vi "Encode.vi"(8 "error in (no error)":errorcluster, 11 "ISO 14443 B DOWN in":refnum<class "ISO 14443 B DOWN.lvclass">) -> (0 "error out":errorcluster, 3 "ISO 14443 B DOWN out":refnum<class "ISO 14443 B DOWN.lvclass">)   [LabVIEW 2019, in "ISO 14443 B DOWN.lvclass"]
uses:
  ISO 14443 B DOWN.lvclass
  TypeDef/Store.ctl
  ISO 14443 B DOWN.lvclass/ISO 14443 B DOWN.ctl
  RFID system.lvclass
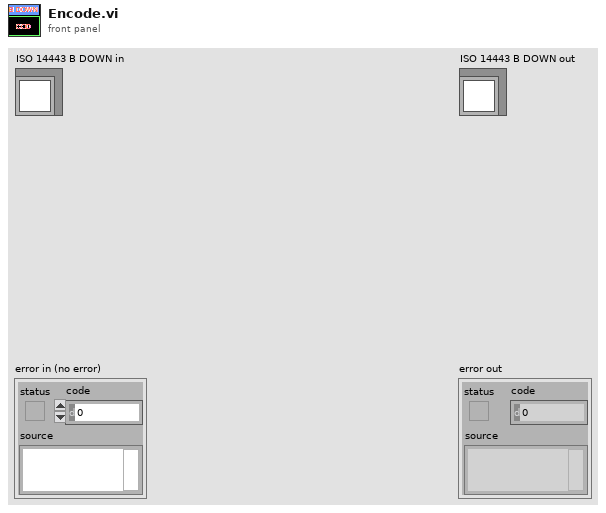
[diagram p1: front panel]
types:
  T1 = typedef "Store.ctl" = enum16{"envelope", "noise", "demSubCar", "CH_frame", "Decode", "demodulate", "in", "out", "sum", "subCarrier", "frame", "command", "encode", "modulate", "encode_UP", "modulate_up", "demod_up", "envelop_up", "sum_up", "out_up", "in_up"}
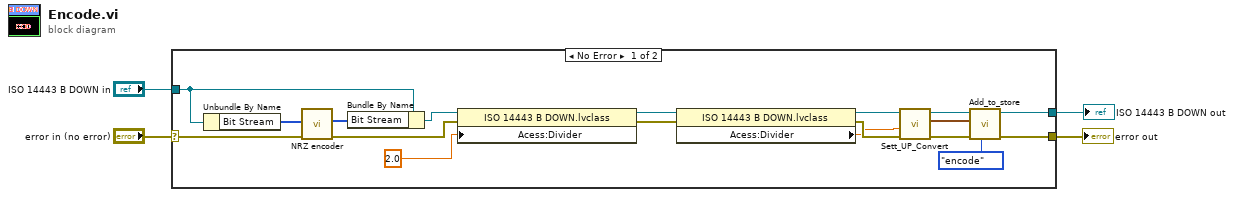
[diagram p0: block diagram]
diagram:
  n1 = case shown="No Error" "error in (no error)" {
    selector: "error in (no error)" -> [w21 w23]
    tunnel: "ISO 14443 B DOWN in" -> [w19 w24]
    tunnel: [w17 w24] -> w2
    tunnel: [w20 w23] -> w1
    frame No Error {
      n2 = Unbundle By Name(w19) -> ("Bit Stream"=w22:u8[])
      n3 = call "NRZ encoder.vi"("Error In"=w21, "Bit stream in"=w22) -> ("error out"=w9:errorcluster, "Bit stream out (NRZ encode)"=w18:u8[])  [unwired: 8 in]
      n4 = Bundle By Name(cluster=w19, "Bit Stream"=w18) -> (w13:refnum<class "ISO 14443 B DOWN.lvclass">)
      n5 = property class="ISO 14443 B DOWN.lvclass"(reference=w13, error in=w9, "Acess:Divider"=2.0 ("Divider(1)")) -> (reference out=w11:refnum<class "ISO 14443 B DOWN.lvclass">, error out=w8:errorcluster)
      n6 = property class="ISO 14443 B DOWN.lvclass"(reference=w11, error in=w8) -> (reference out=w10:refnum<class "ISO 14443 B DOWN.lvclass">, error out=w7:errorcluster, "Acess:Divider"=w6:dbl)
      n7 = call-dynamic "Sett_UP_Convert.vi"("error in (no error)"=w7, "Divider(1)"=w6, "ISO 14443 B DOWN in"=w10) -> ("error out"=w16:errorcluster, "Waveform"=w14:waveform(dbl), "ISO 14443 B DOWN out"=w15:refnum<class "ISO 14443 B DOWN.lvclass">)  [unwired: 6 in]
      n8 = call "Add_to_store.vi"("Store"=Store."encode", "error in (no error)"=w16, "Waveform"=w14, "RFID system in"=w15) -> ("error out"=w20:errorcluster, "RFID system out"=w17:refnum<class "ISO 14443 B DOWN.lvclass">)  [unwired: 6 in]
    }
    frame Error {
    }
  }
  "error out" <- w1
  "ISO 14443 B DOWN out" <- w2
